vi "Initialize.vi"(0 "Pulse Train in":refnum<class "Pulse Train.lvclass">, 1 "Filter in":refnum<class "Filter.lvclass">, 5 "Level in":refnum<class "Level.lvclass">, 7 "Fs (Hz)":dbl, 9 "Npts":i32, 11 "error in (no error)":errorcluster, 13 "Channel Name":string) -> (3 "Filter out":refnum<class "Filter.lvclass">, 4 "Pulse Train out":refnum<class "Pulse Train.lvclass">, 6 "Level out":refnum<class "Level.lvclass">, 15 "error out":errorcluster)   [LabVIEW 2020, in "Pulse Train.lvclass"]
uses:
  Pulse Train.lvclass
  Level/Level.lvclass
  Filter/Filter.lvclass
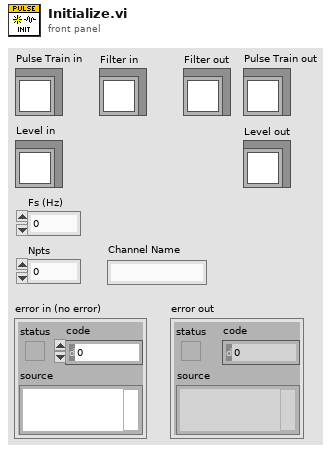
[diagram p1: front panel]
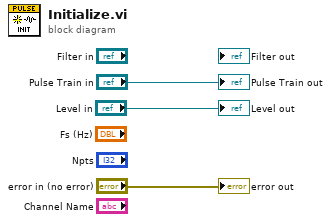
[diagram p0: block diagram]
diagram:
  "error out" <- "error in (no error)"
  "Pulse Train out" <- "Pulse Train in"
  "Level out" <- "Level in"
